vi "solar_app Splash Open.vi"(4 "App Setup":string, 6 "Part Number":string, 7 "SOLAR Version":string, 8 "error in (no error)":errorcluster, 9 "Exe Version":string, 10 "Splash Path (\"\")":string, 11 "Splash msWait (-1)":i32=-1) -> (0 "error out":errorcluster, 3 "Splash VI Refnum":refnum<vi>)   [LabVIEW 2018]
doc: "This opens a splash screen window."
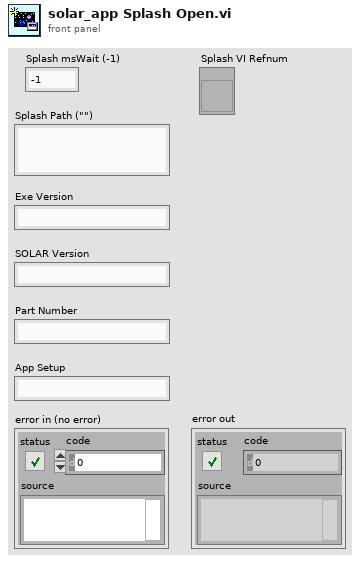
[diagram p1: front panel]
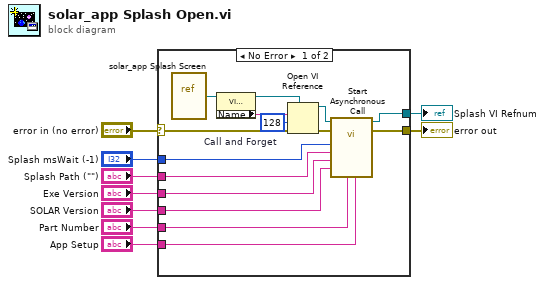
[diagram p0: block diagram]
diagram:
  n1 = case shown="No Error" "error in (no error)" {
    selector: "error in (no error)" -> [w11 w25]
    tunnel: [w24 _] -> w9
    tunnel: "Splash msWait (-1)" -> [w23 _]
    tunnel: "Splash Path (\"\")" -> [w22 _]
    tunnel: "Exe Version" -> [w21 _]
    tunnel: "SOLAR Version" -> [w20 _]
    tunnel: "Part Number" -> [w19 _]
    tunnel: "App Setup" -> [w18 _]
    tunnel: [w10 w25] -> w1
    frame No Error {
      w15 = 128  # Call and Forget
      n2 = vi-ref "solar_app Splash Screen.vi"() -> (w12:refnum<vi>)
      n3 = property class="VI (strict)"(reference=w12) -> (reference out=w13:refnum<vi>, "Name"=w14:string)  [unwired: 1 in, 1 out]
      n4 = Open VI Reference(type specifier VI Refnum (for type only)=w13, vi path=w14, options=w15, error in (no error)=w11) -> (vi reference=w17:refnum<vi>, error out=w16:errorcluster)  [unwired: 2 in]
      n5 = call-by-ref "Start Asynchronous Call"(reference=w17, error in=w16, "AppSetup"=w18, "PartNumber"=w19, "SOLARVersion"=w20, "AppVersion"=w21, "SplashPath"=w22, "SplashWait"=w23) -> (reference out=w24:refnum<vi>, error out=w10:errorcluster)  [unwired: 6 in]
    }
    frame Error {
    }
  }
  "Splash VI Refnum" <- w9
  "error out" <- w1
